vi "Remove Digital Pattern.vi"(8 "error in (no error)":errorcluster, 10 "Page Data in":T1 {"Node Ptr" format="%.0x"}, 11 "State queue in":string[](array[string])) -> (0 "error out":errorcluster, 2 "Page Data out":T1 {"Node Ptr" format="%.0x"}, 3 "State queue out":string[](array[string]))   [LabVIEW 2020, in "Engine Simulation Toolkit System Explorer.lvlib"]
uses:
  Engine Simulation Toolkit System Explorer.lvlib
  Digital Patterns Page Data.ctl
  <vilib>/NI VeriStand/Custom Device API/Custom Device Item Ref.ctl
  Digital Pattern.ctl
  Digital Pattern Base.ctl
  Digital Pattern Remove Edge.ctl
  Digital Pattern Add Pulse.ctl
  <vilib>/NI VeriStand/Custom Device API/Custom Device API.lvlib
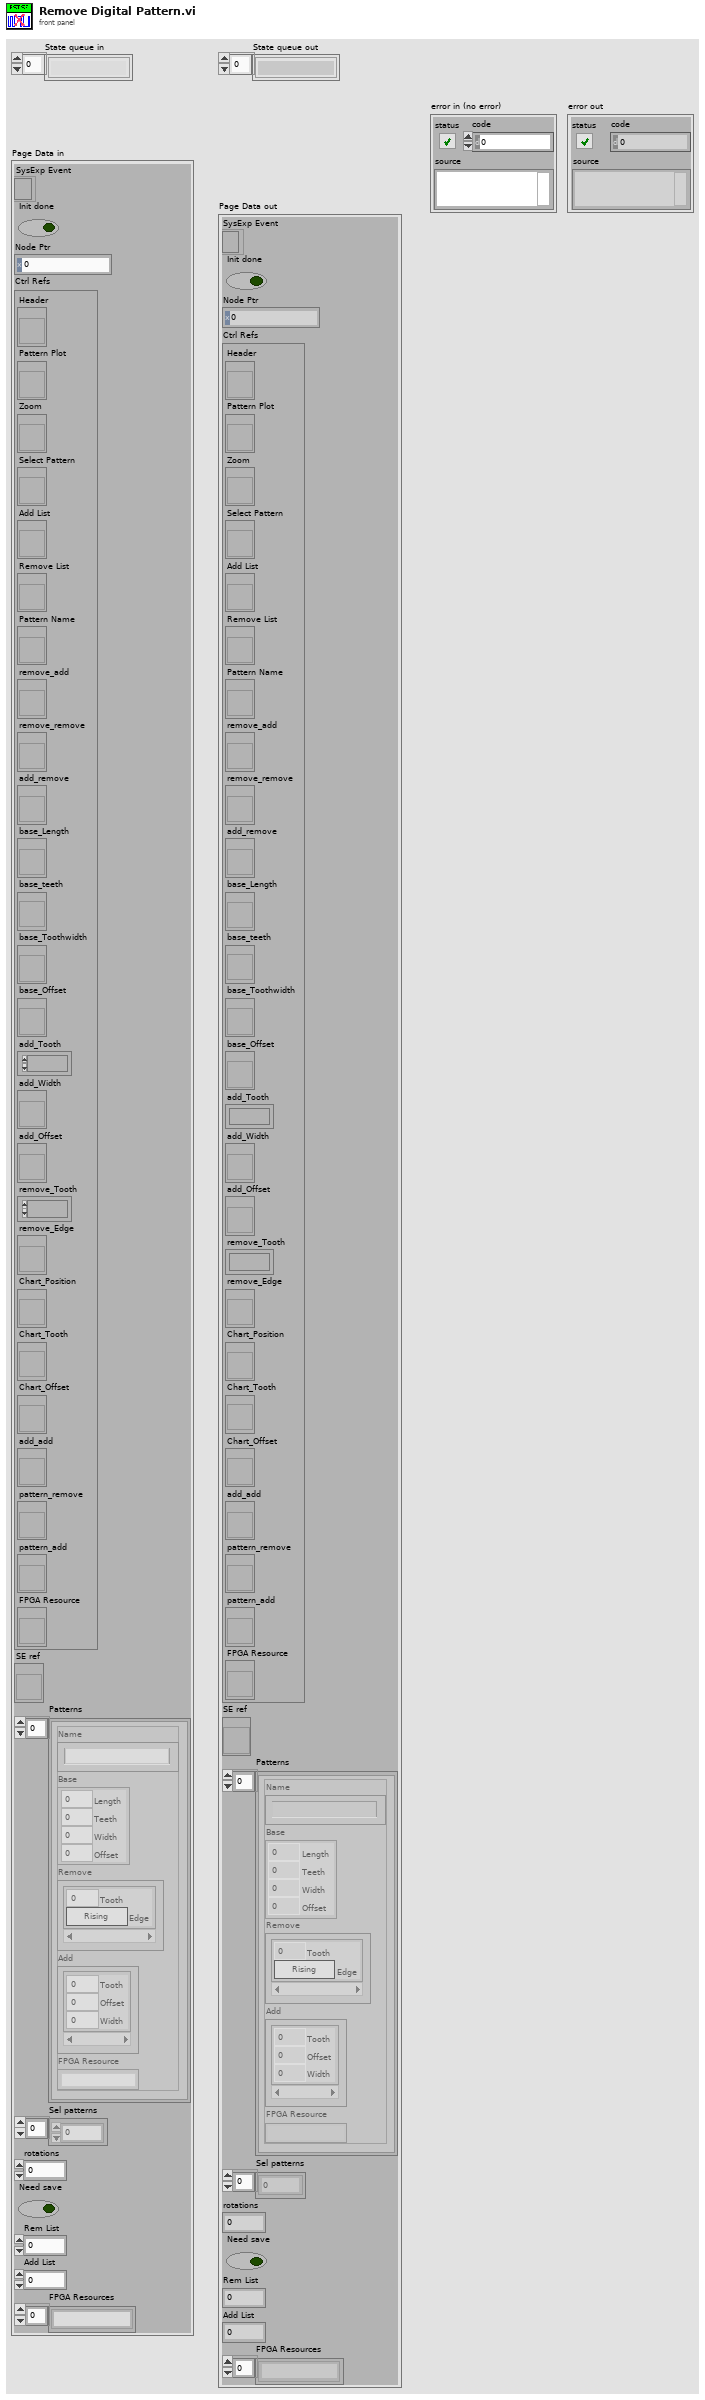
[diagram p1: front panel]
types:
  T1 = typedef "Engine Simulation Toolkit System Explorer.lvlib/Digital Patterns Page Data.ctl" = cluster{"SysExp Event":refnum<event-registration>, "Init done":bool, "Node Ptr":T2, "Ctrl Refs":cluster{"Header":refnum<vi>, "Pattern Plot":refnum<vi>, "Zoom":refnum<vi>, "Select Pattern":refnum<vi>, "Add List":refnum<vi>, "Remove List":refnum<vi>, "Pattern Name":refnum<vi>, "remove_add":refnum<vi>, "remove_remove":refnum<vi>, "add_remove":refnum<vi>, "base_Length":refnum<vi>, "base_teeth":refnum<vi>, "base_Toothwidth":refnum<vi>, "base_Offset":refnum<vi>, "add_Tooth":refnum<vi>, "add_Width":refnum<vi>, "add_Offset":refnum<vi>, "remove_Tooth":refnum<vi>, "remove_Edge":refnum<vi>, "Chart_Position":refnum<vi>, "Chart_Tooth":refnum<vi>, "Chart_Offset":refnum<vi>, "add_add":refnum<vi>, "pattern_remove":refnum<vi>, "pattern_add":refnum<vi>, "FPGA Resource":refnum<vi>}, "SE ref":refnum<vi>, "Patterns":T3[], "Sel patterns":i32[], "rotations":u16, "Need save":bool, "Rem List":i32, "Add List":i32, "FPGA Resources":string[]}
  T2 = typedef "Custom Device API.lvlib/Custom Device Item Ref.ctl" = u64
  T3 = typedef "Engine Simulation Toolkit System Explorer.lvlib/Digital Pattern.ctl" = cluster{"Name":string, "Base":T4, "Remove":T5[], "Add":T6[], "FPGA Resource":string}
  T4 = typedef "Engine Simulation Toolkit System Explorer.lvlib/Digital Pattern Base.ctl" = cluster{"Length":dbl, "Teeth":u16, "Width":dbl, "Offset":dbl}
  T5 = typedef "Engine Simulation Toolkit System Explorer.lvlib/Digital Pattern Remove Edge.ctl" = cluster{"Tooth":u16, "Edge":bool}
  T6 = typedef "Engine Simulation Toolkit System Explorer.lvlib/Digital Pattern Add Pulse.ctl" = cluster{"Tooth":u16, "Offset":dbl, "Width":dbl}
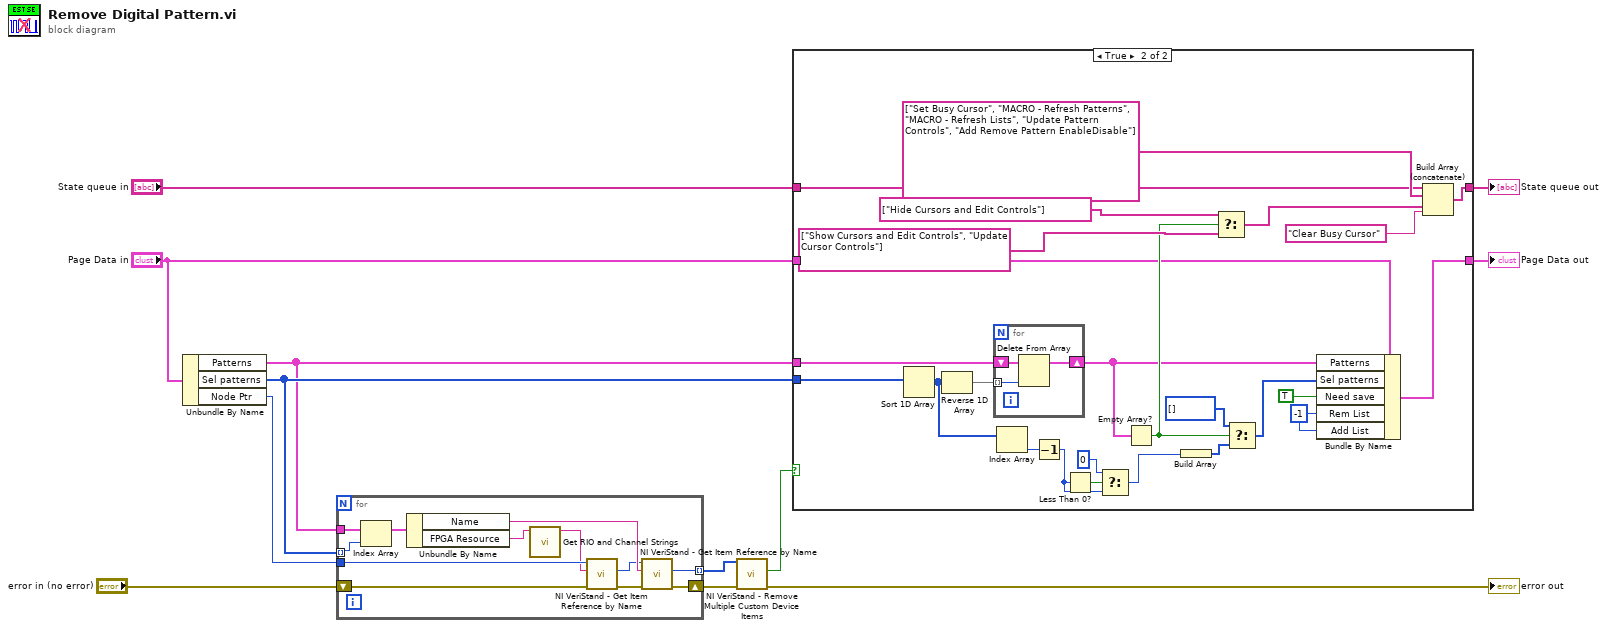
[diagram p0: block diagram]
diagram:
  n1 = Unbundle By Name("Page Data in") -> ("Patterns"=w6:T3[], "Sel patterns"=w7:i32[], "Node Ptr"=w5:T2)
  n2 = for {
    tunnel: w7 -> [w22] mode=indexing
    tunnel: w6 -> [w24]
    tunnel: w5 -> [w17]
    tunnel: [w20] -> w3 mode=indexing
    shift-right: [w19] -> w4
    shift-left: "error in (no error)" -> [w15]
    n3 = Index Array(array=w24, index=w22) -> (element=w23:T3)
    n4 = Unbundle By Name(w23) -> ("Name"=w21:string, "FPGA Resource"=w18:string)
    n5 = call "Get RIO and Channel Strings.vi"("rio/channel"=w18) -> ("rio"=w13:string)  [unwired: 9 in, 1 out]
    n6 = call <vilib>:"NI VeriStand - Get Item Reference by Name.vi"("error in (no error)"=w15, "Item Name"=w13, "Parent Ref in"=w17) -> ("error out"=w14:errorcluster, "Item Ref"=w16:T2)  [unwired: 5 in, 2 out]
    n7 = call <vilib>:"NI VeriStand - Get Item Reference by Name.vi"("error in (no error)"=w14, "Item Name"=w21, "Parent Ref in"=w16) -> ("error out"=w19:errorcluster, "Item Ref"=w20:T2)  [unwired: 5 in, 2 out]
  }
  n8 = call <vilib>:"NI VeriStand - Remove Multiple Custom Device Items.vi"("error in (no error)"=w4, "Item Refs in"=w3) -> ("error out"=→"error out":errorcluster, "Deleted?"=w2:bool)  [unwired: 8 in]
  n9 = case shown="True" w2 {
    tunnel: [w26 w34] -> w12
    tunnel: [w25 w32] -> w11
    tunnel: "Page Data in" -> [w25 w31]
    tunnel: "State queue in" -> [w26 w30]
    tunnel: w7 -> [_ w28]
    tunnel: w6 -> [_ w27]
    frame False {
    }
    frame True {
      w40 = -1 ("Rem List")
      n10 = Sort 1D Array(array=w28) -> (sorted array=w41:i32[])
      n11 = Reverse 1D Array(array=w41) -> (reversed array=w29:i32[])
      n12 = for {
        tunnel: w29 -> [w54] mode=indexing
        shift-right: [w53] -> w35
        shift-left: w27 -> [w52]
        n13 = Delete From Array(array=w52, index=w54) -> (array with subset deleted=w53:T3[])  [unwired: 1 in, 1 out]
      }
      n14 = Index Array(array=w41) -> (element=w38:i32)  [unwired: 1 in]
      n15 = Decrement(x=w38) -> (x-1=w43:i32)
      n16 = Less Than 0?(x=w43) -> (x < 0?=w42:bool)
      n17 = Select(t=0, s=w42, f=w43) -> (s? t:f=w44:i32)
      n18 = Empty Array?(array=w35) -> (empty?=w47:bool)
      n19 = Build Array(w44) -> (w39:i32[])
      n20 = Select(t=string[] ["Hide Cursors and Edit Controls"], s=w47, f=string[] ["Show Cursors and Edit Controls", "Update Cursor Controls"]) -> (s? t:f=w48:string[])
      n21 = Select(t=i32[] [] ("appended array"), s=w47, f=w39) -> (s? t:f=w37:i32[])
      n22 = Bundle By Name(cluster=w31, "Patterns"=w35, "Sel patterns"=w37, "Need save"=TRUE, "Rem List"=w40, "Add List"=w40) -> (w32:T1)
      n23 = Build Array (concatenate)(w30, string[] ["Set Busy Cursor", "MACRO - Refresh Patterns", "MACRO - Refresh Lists", "Update Pattern Controls", "Add Remove Pattern EnableDisable"], w48, "Clear Busy Cursor") -> (w34:string[])
    }
  }
  "State queue out" <- w12
  "Page Data out" <- w11
